vi "Githubtest.vi"() -> ()   [LabVIEW 2013]
panel:
  in  "Slide":dbl(slide) scale=0.0..10.0
  out "Gauge":dbl(knob) scale=0.0..10.0
  out "Boolean 2":bool
  in  "Boolean":bool
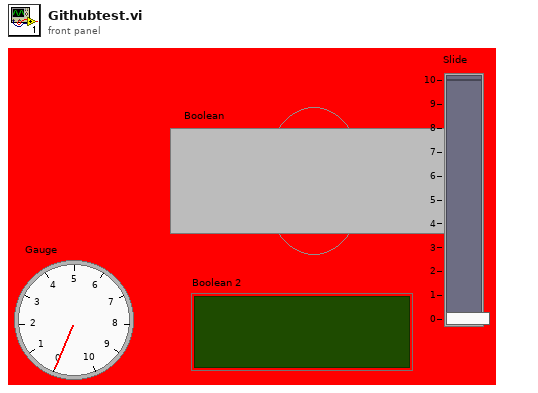
[diagram p1: front panel]
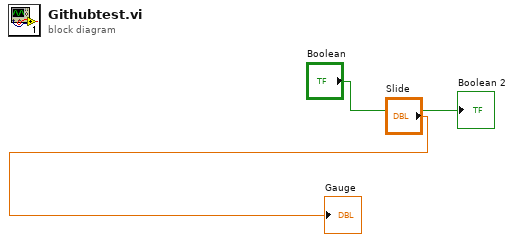
[diagram p0: block diagram]
diagram:
  "Boolean 2" <- "Boolean"
  "Gauge" <- "Slide"
